vi "myRIO_BRig_RT__Case_Exp_State_initTrial_LC_Sel__v3.vi"(6 "input_dataTrial":u16[][](array[numeric]), 7 "input_spout":enum16{"Left", "Right"}(ring), 8 "input_arrTrig":bool[](array[boolean]), 9 "input_dataBlock":u16[][](array[numeric]), 10 "input_dataLC":u16[](array[numeric]), 11 "input_dataCurrent":u16[](array[numeric])) -> (0 "output_arrTrig":bool[](array[boolean]), 4 "output_dataTrial":u16[][](array[numeric]), 5 "output_dataCurrent":u16[](array[numeric]))   [LabVIEW 2014]
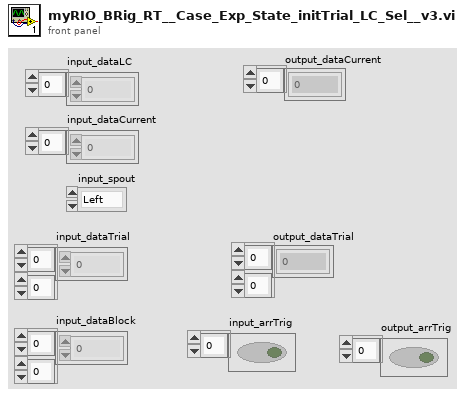
[diagram p1: front panel]
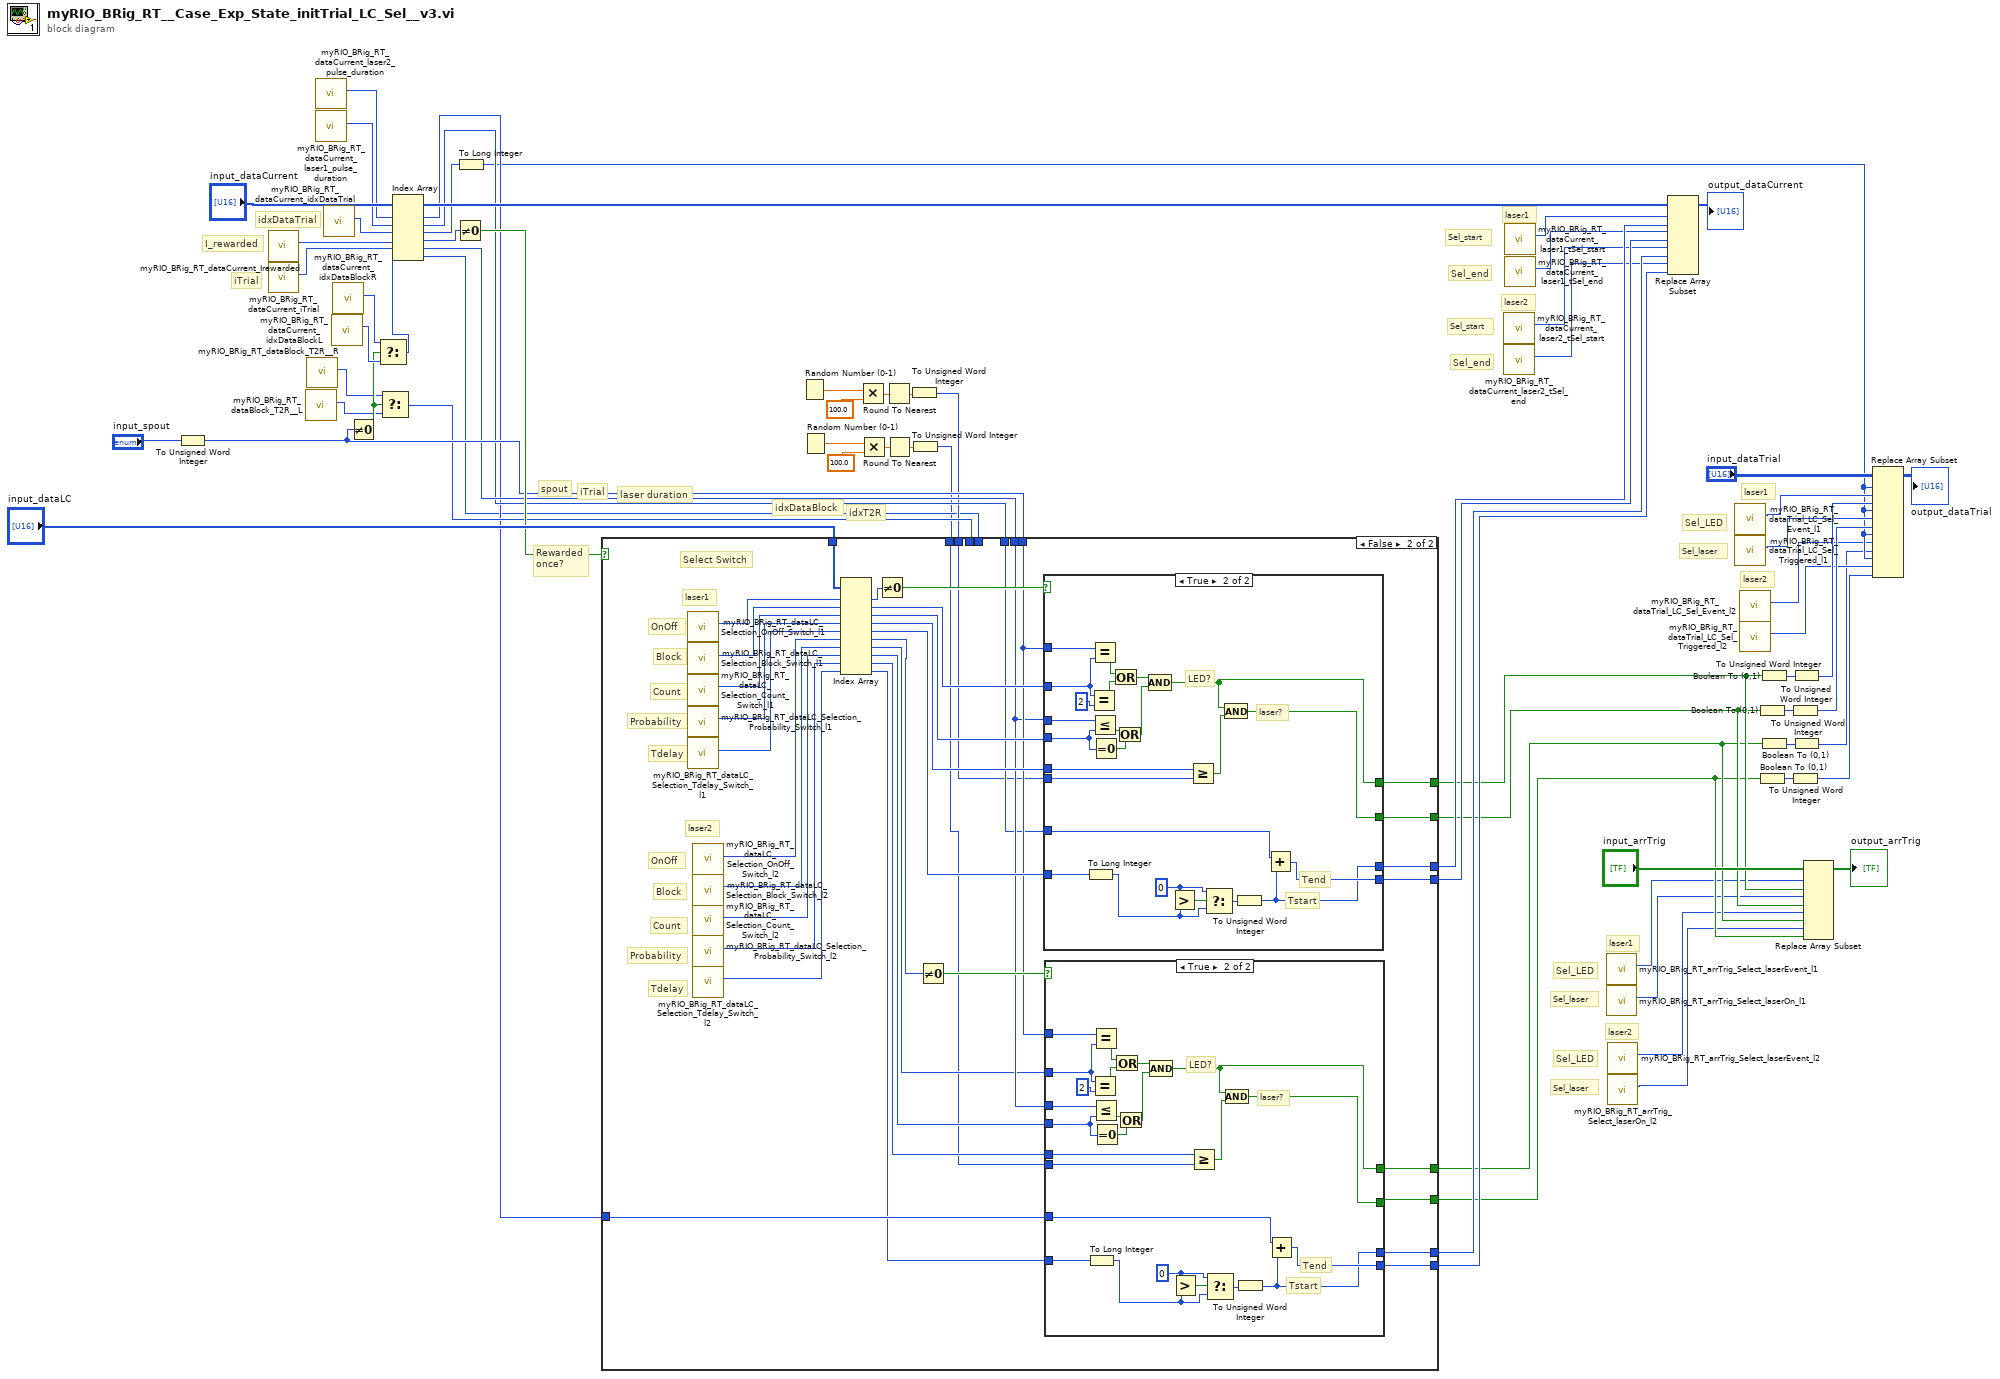
[diagram p0: block diagram]
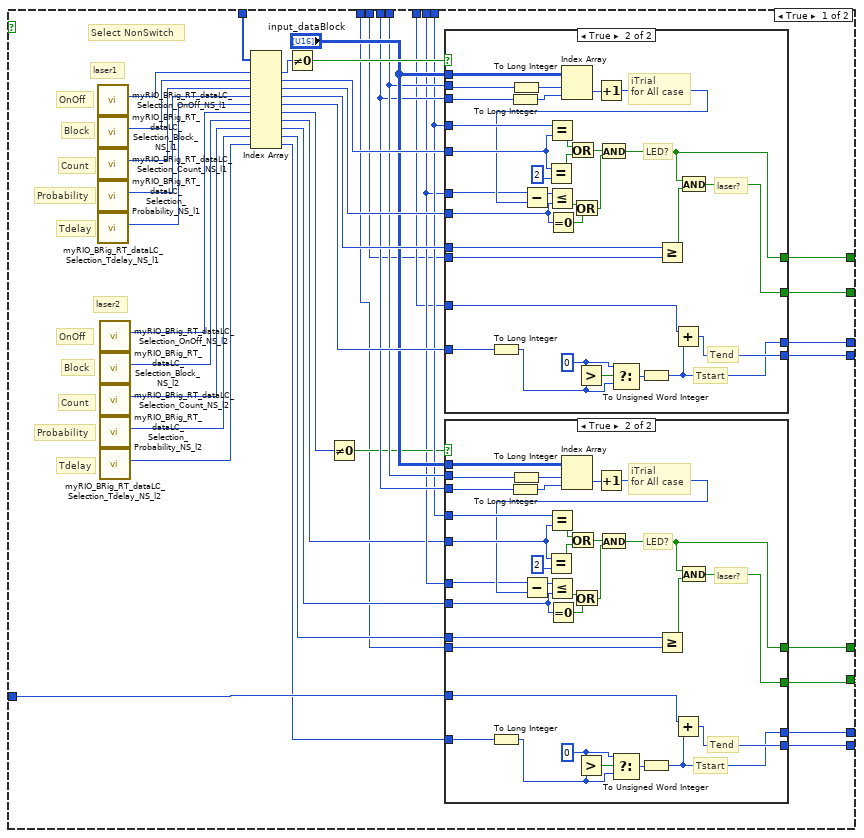
[diagram p2: hidden frame]
diagram:
  # "Sel_LED"
  # "Sel_laser"
  # "Sel_end"
  # "Sel_start"
  # "Sel_LED"
  # "Sel_laser"
  # "Sel_end"
  # "Sel_start"
  # "Sel_LED"
  # "Sel_laser"
  # "laser2"
  # "laser1"
  # "laser2"
  # "laser1"
  # "laser2"
  # "laser1"
  # "idxT2R"
  # "idxDataBlock"
  # "laser duration"
  # "iTrial"
  # "spout"
  # "Rewarded\nonce?"
  # "iTrial"
  # "idxDataTrial"
  # "I_rewarded"
  n1 = To Unsigned Word Integer(number="input_spout") -> (unsigned 16bit integer=w43:u16)
  n2 = call "myRIO_BRig_RT_dataCurrent_Irewarded.vi"() -> ("output_I_rewarded"=w65:i32)  [unwired: 11 in]
  n3 = call "myRIO_BRig_RT_dataCurrent_iTrial.vi"() -> ("output_iTrial"=w54:i32)  [unwired: 11 in]
  n4 = call "myRIO_BRig_RT_dataBlock_T2R__L.vi"() -> ("output_T2R__L"=w49:i32)  [unwired: 11 in]
  n5 = call "myRIO_BRig_RT_dataBlock_T2R__R.vi"() -> ("output_T2R__R"=w50:i32)  [unwired: 11 in]
  n6 = call "myRIO_BRig_RT_dataCurrent_laser2_pulse_duration.vi"() -> ("output_laser2_pulse_duration"=w24:i32)  [unwired: 11 in]
  n7 = call "myRIO_BRig_RT_dataCurrent_laser1_pulse_duration.vi"() -> ("output_laser1_pulse_duration"=w48:i32)  [unwired: 11 in]
  n8 = call "myRIO_BRig_RT_dataCurrent_idxDataTrial.vi"() -> ("output_idxDataTrial"=w58:i32)  [unwired: 11 in]
  n9 = call "myRIO_BRig_RT_dataCurrent_idxDataBlockL.vi"() -> ("output_idxDataBlock__L"=w53:i32)  [unwired: 11 in]
  n10 = call "myRIO_BRig_RT_dataCurrent_idxDataBlockR.vi"() -> ("output_idxDataBlock__R"=w52:i32)  [unwired: 11 in]
  n11 = Not Equal To 0?(x=w43) -> (x != 0?=w51:bool)
  n12 = Select(t=w52, s=w51, f=w53) -> (s? t:f=w21:i32)
  n13 = Select(t=w50, s=w51, f=w49) -> (s? t:f=w40:i32)
  n14 = Index Array(array="input_dataCurrent", index #1=w24, index #2=w48, index #3=w58, index #4=w65, index #5=w54, index #6=w21) -> (element #1=w23:u16, element #2=w41:u16, element #3=w57:u16, element #4=w66:u16, element #5=w42:u16, element #6=w22:u16)
  n15 = Not Equal To 0?(x=w66) -> (x != 0?=w44:bool)
  n16 = To Long Integer(number=w57) -> (32bit integer=w10:i32)
  n17 = Random Number (0-1)() -> (number: 0 to 1=w36:dbl)
  n18 = Random Number (0-1)() -> (number: 0 to 1=w2:dbl)
  n19 = Multiply(x=w36, y=100.0) -> (x*y=w37:dbl)
  n20 = Multiply(x=w2, y=100.0) -> (x*y=w3:dbl)
  n21 = Round To Nearest(number=w37) -> (nearest integer value=w38:dbl)
  n22 = Round To Nearest(number=w3) -> (nearest integer value=w4:dbl)
  n23 = To Unsigned Word Integer(number=w38) -> (unsigned 16bit integer=w35:u16)
  n24 = To Unsigned Word Integer(number=w4) -> (unsigned 16bit integer=w1:u16)
  n25 = case shown="False" w44 {
    tunnel: "input_dataLC" -> [w107 w208]
    tunnel: w43 -> [w97 w192]
    tunnel: w42 -> [w95 w191]
    tunnel: w41 -> [w94 w190]
    tunnel: w22 -> [w99 _]
    tunnel: w40 -> [w98 _]
    tunnel: w35 -> [w68 w172]
    tunnel: [w93 w201] -> w28
    tunnel: [w92 w200] -> w27
    tunnel: [w91 w199] -> w34
    tunnel: [w90 w198] -> w33
    tunnel: [w89 w196] -> w26
    tunnel: [w88 w195] -> w25
    tunnel: [w87 w194] -> w32
    tunnel: [w86 w193] -> w31
    tunnel: w23 -> [w85 w189]
    tunnel: w1 -> [w69 w173]
    frame True {
      # "laser2"
      # "laser1"
      # "Count"
      # "Tdelay"
      # "Probability"
      # "OnOff"
      # "Block"
      # "Count"
      # "Tdelay"
      # "Probability"
      # "OnOff"
      # "Block"
      # "Select NonSwitch"
      n26 = call "myRIO_BRig_RT_dataLC_Selection_OnOff_NS_l1.vi"() -> ("output_Selection_OnOff_NS_l1"=w70:i32)  [unwired: 11 in]
      n27 = call "myRIO_BRig_RT_dataLC_Selection_Block_NS_l1.vi"() -> ("output_Selection_Block_NS_l1"=w71:i32)  [unwired: 11 in]
      n28 = call "myRIO_BRig_RT_dataLC_Selection_Count_NS_l1.vi"() -> ("output_Selection_Count_NS_l1"=w72:i32)  [unwired: 11 in]
      n29 = call "myRIO_BRig_RT_dataLC_Selection_Probability_NS_l1.vi"() -> ("output_Selection_Probability_NS_l1"=w73:i32)  [unwired: 11 in]
      n30 = call "myRIO_BRig_RT_dataLC_Selection_Tdelay_NS_l1.vi"() -> ("output_Selection_Tdelay_NS_l1"=w74:i32)  [unwired: 11 in]
      n31 = call "myRIO_BRig_RT_dataLC_Selection_OnOff_NS_l2.vi"() -> ("output_Selection_OnOff_NS_l2"=w79:i32)  [unwired: 11 in]
      n32 = call "myRIO_BRig_RT_dataLC_Selection_Block_NS_l2.vi"() -> ("output_Selection_Block_NS_l2"=w78:i32)  [unwired: 11 in]
      n33 = call "myRIO_BRig_RT_dataLC_Selection_Count_NS_l2.vi"() -> ("output_Selection_Count_NS_l2"=w77:i32)  [unwired: 11 in]
      n34 = call "myRIO_BRig_RT_dataLC_Selection_Probability_NS_l2.vi"() -> ("output_Selection_Probability_NS_l2"=w76:i32)  [unwired: 11 in]
      n35 = call "myRIO_BRig_RT_dataLC_Selection_Tdelay_NS_l2.vi"() -> ("output_Selection_Tdelay_NS_l2"=w75:i32)  [unwired: 11 in]
      n36 = Index Array(array=w107, index #1=w70, index #2=w71, index #3=w72, index #4=w73, index #5=w74, index #6=w79, index #7=w78, index #8=w77, index #9=w76, index #10=w75) -> (element #1=w103:u16, element #2=w101:u16, element #3=w106:u16, element #4=w105:u16, element #5=w104:u16, element #6=w84:u16, element #7=w83:u16, element #8=w82:u16, element #9=w81:u16, element #10=w80:u16)
      n37 = Not Equal To 0?(x=w103) -> (x != 0?=w102:bool)
      n38 = Not Equal To 0?(x=w84) -> (x != 0?=w96:bool)
      n39 = case shown="True" w102 {
        tunnel: w97 -> [_ w170]
        tunnel: w95 -> [_ w155]
        tunnel: [_ w150] -> w93
        tunnel: [_ w166] -> w92
        tunnel: [_ w146] -> w90
        tunnel: [_ w145] -> w91
        tunnel: w94 -> [_ w144]
        tunnel: w98 -> [_ w161]
        tunnel: w99 -> [_ w163]
        tunnel: w101 -> [_ w158]
        tunnel: w106 -> [_ w157]
        tunnel: w105 -> [_ w153]
        tunnel: w104 -> [_ w143]
        tunnel: "input_dataBlock" -> [_ w142]
        tunnel: w68 -> [_ w141]
        frame False {
        }
        frame True {
          w148 = 0 ("x")
          # "Tstart"
          # "Tend"
          # "iTrial\nfor All case"
          # "laser?"
          # "LED?"
          n40 = To Long Integer(number=w143) -> (32bit integer=w140:i32)
          n41 = To Long Integer(number=w161) -> (32bit integer=w160:i32)
          n42 = To Long Integer(number=w163) -> (32bit integer=w162:i32)
          n43 = Equal?(x=w158, y=u16 2) -> (x = y?=w168:bool)
          n44 = Equal?(x=w170, y=w158) -> (x = y?=w169:bool)
          n45 = Equal To 0?(x=w157) -> (x = 0?=w164:bool)
          n46 = Index Array(array=w142, index (row)=w162, index (col)=w160) -> (element=w159:u16)
          n47 = Or(x=w169, y=w168) -> (x .or. y?=w152:bool)
          n48 = Greater?(x=w148, y=w140) -> (0:w147:bool)
          n49 = Increment(x=w159) -> (x+1=w156:u16)
          n50 = Subtract(x=w155, y=w156) -> (x-y=w154:u16)
          n51 = Less Or Equal?(x=w154, y=w157) -> (x <= y?=w165:bool)
          n52 = Or(x=w165, y=w164) -> (x .or. y?=w151:bool)
          n53 = And(x=w152, y=w151) -> (x .and. y?=w150:bool)
          n54 = Select(t=w148, s=w147, f=w140) -> (s? t:f=w149:i32)
          n55 = To Unsigned Word Integer(number=w149) -> (unsigned 16bit integer=w145:u16)
          n56 = Greater Or Equal?(x=w153, y=w141) -> (x >= y?=w167:bool)
          n57 = Add(x=w144, y=w145) -> (x+y=w146:u16)
          n58 = And(x=w150, y=w167) -> (x .and. y?=w166:bool)
        }
      }
      n59 = case shown="True" w96 {
        tunnel: w97 -> [_ w138]
        tunnel: w95 -> [_ w123]
        tunnel: [_ w118] -> w89
        tunnel: [_ w134] -> w88
        tunnel: [_ w114] -> w86
        tunnel: [_ w113] -> w87
        tunnel: w85 -> [_ w112]
        tunnel: w98 -> [_ w129]
        tunnel: w99 -> [_ w131]
        tunnel: w83 -> [_ w126]
        tunnel: w82 -> [_ w125]
        tunnel: w81 -> [_ w121]
        tunnel: w80 -> [_ w111]
        tunnel: "input_dataBlock" -> [_ w110]
        tunnel: w69 -> [_ w109]
        frame False {
        }
        frame True {
          w116 = 0 ("x")
          # "Tstart"
          # "Tend"
          # "iTrial\nfor All case"
          # "laser?"
          # "LED?"
          n60 = To Long Integer(number=w111) -> (32bit integer=w108:i32)
          n61 = To Long Integer(number=w129) -> (32bit integer=w128:i32)
          n62 = To Long Integer(number=w131) -> (32bit integer=w130:i32)
          n63 = Equal?(x=w126, y=u16 2) -> (x = y?=w136:bool)
          n64 = Equal?(x=w138, y=w126) -> (x = y?=w137:bool)
          n65 = Equal To 0?(x=w125) -> (x = 0?=w132:bool)
          n66 = Index Array(array=w110, index (row)=w130, index (col)=w128) -> (element=w127:u16)
          n67 = Or(x=w137, y=w136) -> (x .or. y?=w120:bool)
          n68 = Greater?(x=w116, y=w108) -> (0:w115:bool)
          n69 = Increment(x=w127) -> (x+1=w124:u16)
          n70 = Subtract(x=w123, y=w124) -> (x-y=w122:u16)
          n71 = Less Or Equal?(x=w122, y=w125) -> (x <= y?=w133:bool)
          n72 = Or(x=w133, y=w132) -> (x .or. y?=w119:bool)
          n73 = And(x=w120, y=w119) -> (x .and. y?=w118:bool)
          n74 = Select(t=w116, s=w115, f=w108) -> (s? t:f=w117:i32)
          n75 = To Unsigned Word Integer(number=w117) -> (unsigned 16bit integer=w113:u16)
          n76 = Greater Or Equal?(x=w121, y=w109) -> (x >= y?=w135:bool)
          n77 = Add(x=w112, y=w113) -> (x+y=w114:u16)
          n78 = And(x=w118, y=w135) -> (x .and. y?=w134:bool)
        }
      }
    }
    frame False {
      # "laser2"
      # "laser1"
      # "Count"
      # "Tdelay"
      # "Probability"
      # "OnOff"
      # "Block"
      # "Count"
      # "Tdelay"
      # "Probability"
      # "OnOff"
      # "Block"
      # "Select Switch"
      n79 = call "myRIO_BRig_RT_dataLC_Selection_OnOff_Switch_l1.vi"() -> ("output_Selection_OnOff_Switch_l1"=w188:i32)  [unwired: 11 in]
      n80 = call "myRIO_BRig_RT_dataLC_Selection_Block_Switch_l1.vi"() -> ("output_Selection_Block_Switch_l1"=w187:i32)  [unwired: 11 in]
      n81 = call "myRIO_BRig_RT_dataLC_Selection_Count_Switch_l1.vi"() -> ("output_Selection_Count_Switch_l1"=w186:i32)  [unwired: 11 in]
      n82 = call "myRIO_BRig_RT_dataLC_Selection_Probability_Switch_l1.vi"() -> ("output_Selection_Probability_Switch_l1"=w185:i32)  [unwired: 11 in]
      n83 = call "myRIO_BRig_RT_dataLC_Selection_Tdelay_Switch_l1.vi"() -> ("output_Selection_Tdelay_Switch_l1"=w184:i32)  [unwired: 11 in]
      n84 = call "myRIO_BRig_RT_dataLC_Selection_OnOff_Switch_l2.vi"() -> ("output_Selection_OnOff_Switch_l2"=w174:i32)  [unwired: 11 in]
      n85 = call "myRIO_BRig_RT_dataLC_Selection_Block_Switch_l2.vi"() -> ("output_Selection_Block_Switch_l2"=w175:i32)  [unwired: 11 in]
      n86 = call "myRIO_BRig_RT_dataLC_Selection_Count_Switch_l2.vi"() -> ("output_Selection_Count_Switch_l2"=w176:i32)  [unwired: 11 in]
      n87 = call "myRIO_BRig_RT_dataLC_Selection_Probability_Switch_l2.vi"() -> ("output_Selection_Probability_Switch_l1"=w177:i32)  [unwired: 11 in]
      n88 = call "myRIO_BRig_RT_dataLC_Selection_Tdelay_Switch_l2.vi"() -> ("output_Selection_Tdelay_Switch_l2"=w178:i32)  [unwired: 11 in]
      n89 = Index Array(array=w208, index #1=w188, index #2=w187, index #3=w186, index #4=w185, index #5=w184, index #6=w174, index #7=w175, index #8=w176, index #9=w177, index #10=w178) -> (element #1=w207:u16, element #2=w204:u16, element #3=w203:u16, element #4=w205:u16, element #5=w202:u16, element #6=w183:u16, element #7=w182:u16, element #8=w181:u16, element #9=w180:u16, element #10=w179:u16)
      n90 = Not Equal To 0?(x=w207) -> (x != 0?=w206:bool)
      n91 = Not Equal To 0?(x=w183) -> (x != 0?=w197:bool)
      n92 = case shown="True" w206 {
        tunnel: w192 -> [_ w255]
        tunnel: w204 -> [_ w254]
        tunnel: w191 -> [_ w253]
        tunnel: [_ w248] -> w201
        tunnel: [_ w247] -> w200
        tunnel: [_ w237] -> w198
        tunnel: w202 -> [_ w239]
        tunnel: [_ w236] -> w199
        tunnel: w203 -> [_ w246]
        tunnel: w190 -> [_ w238]
        tunnel: w172 -> [_ w235]
        tunnel: w205 -> [_ w234]
        frame False {
        }
        frame True {
          w241 = 0 ("x")
          # "Tstart"
          # "Tend"
          # "laser?"
          # "LED?"
          n93 = To Long Integer(number=w239) -> (32bit integer=w233:i32)
          n94 = Equal?(x=w254, y=u16 2) -> (x = y?=w251:bool)
          n95 = Equal?(x=w255, y=w254) -> (x = y?=w252:bool)
          n96 = Less Or Equal?(x=w253, y=w246) -> (x <= y?=w245:bool)
          n97 = Equal To 0?(x=w246) -> (x = 0?=w244:bool)
          n98 = Or(x=w252, y=w251) -> (x .or. y?=w250:bool)
          n99 = Or(x=w245, y=w244) -> (x .or. y?=w243:bool)
          n100 = Compound Arithmetic op=AND(w250, w243) -> (w248:bool)
          n101 = Greater?(x=w241, y=w233) -> (0:w240:bool)
          n102 = Greater Or Equal?(x=w234, y=w235) -> (x >= y?=w249:bool)
          n103 = Select(t=w241, s=w240, f=w233) -> (s? t:f=w242:i32)
          n104 = And(x=w248, y=w249) -> (x .and. y?=w247:bool)
          n105 = To Unsigned Word Integer(number=w242) -> (unsigned 16bit integer=w236:u16)
          n106 = Add(x=w238, y=w236) -> (x+y=w237:u16)
        }
      }
      n107 = case shown="True" w197 {
        tunnel: w192 -> [_ w231]
        tunnel: w182 -> [_ w230]
        tunnel: w191 -> [_ w229]
        tunnel: [_ w224] -> w196
        tunnel: [_ w223] -> w195
        tunnel: [_ w213] -> w193
        tunnel: w179 -> [_ w215]
        tunnel: [_ w212] -> w194
        tunnel: w181 -> [_ w222]
        tunnel: w189 -> [_ w214]
        tunnel: w173 -> [_ w211]
        tunnel: w180 -> [_ w210]
        frame False {
        }
        frame True {
          w217 = 0 ("x")
          # "Tstart"
          # "Tend"
          # "laser?"
          # "LED?"
          n108 = To Long Integer(number=w215) -> (32bit integer=w209:i32)
          n109 = Equal?(x=w230, y=u16 2) -> (x = y?=w227:bool)
          n110 = Equal?(x=w231, y=w230) -> (x = y?=w228:bool)
          n111 = Less Or Equal?(x=w229, y=w222) -> (x <= y?=w221:bool)
          n112 = Equal To 0?(x=w222) -> (x = 0?=w220:bool)
          n113 = Or(x=w228, y=w227) -> (x .or. y?=w226:bool)
          n114 = Or(x=w221, y=w220) -> (x .or. y?=w219:bool)
          n115 = Compound Arithmetic op=AND(w226, w219) -> (w224:bool)
          n116 = Greater?(x=w217, y=w209) -> (0:w216:bool)
          n117 = Greater Or Equal?(x=w210, y=w211) -> (x >= y?=w225:bool)
          n118 = Select(t=w217, s=w216, f=w209) -> (s? t:f=w218:i32)
          n119 = And(x=w224, y=w225) -> (x .and. y?=w223:bool)
          n120 = To Unsigned Word Integer(number=w218) -> (unsigned 16bit integer=w212:u16)
          n121 = Add(x=w214, y=w212) -> (x+y=w213:u16)
        }
      }
    }
  }
  n122 = call "myRIO_BRig_RT_dataCurrent_laser2_tSel_start.vi"() -> ("output_laser2_tSel_start"=w18:i32)  [unwired: 11 in]
  n123 = call "myRIO_BRig_RT_dataCurrent_laser2_tSel_end.vi"() -> ("output_laser2_tSel_end"=w17:i32)  [unwired: 11 in]
  n124 = call "myRIO_BRig_RT_dataCurrent_laser1_tSel_start.vi"() -> ("output_laser1_tSel_start"=w19:i32)  [unwired: 11 in]
  n125 = call "myRIO_BRig_RT_dataCurrent_laser1_tSel_end.vi"() -> ("output_laser1_tSel_end"=w20:i32)  [unwired: 11 in]
  n126 = call "myRIO_BRig_RT_arrTrig_Select_laserEvent_l1.vi"() -> ("output_arrTrig_Select_laserEvent_l1"=w15:i32)  [unwired: 11 in]
  n127 = call "myRIO_BRig_RT_arrTrig_Select_laserOn_l1.vi"() -> ("output_arrTrig_Select_laserOn_l1"=w16:i32)  [unwired: 11 in]
  n128 = call "myRIO_BRig_RT_arrTrig_Select_laserEvent_l2.vi"() -> ("output_arrTrig_Select_laserEvent_l2"=w14:i32)  [unwired: 11 in]
  n129 = call "myRIO_BRig_RT_arrTrig_Select_laserOn_l2.vi"() -> ("output_arrTrig_Select_laserOn_l2"=w13:i32)  [unwired: 11 in]
  n130 = Replace Array Subset(array="input_dataCurrent", new element #1=w34, index #1=w19, new element #2=w33, index #2=w20, new element #3=w32, index #3=w18, new element #4=w31, index #4=w17) -> (→"output_dataCurrent":u16[])
  n131 = call "myRIO_BRig_RT_dataTrial_LC_Sel_Event_l1.vi"() -> ("output_LC_Sel_Event_l1"=w11:i32)  [unwired: 11 in]
  n132 = call "myRIO_BRig_RT_dataTrial_LC_Sel_Triggered_l1.vi"() -> ("output_LC_Sel_Triggered_l1"=w12:i32)  [unwired: 11 in]
  n133 = call "myRIO_BRig_RT_dataTrial_LC_Sel_Event_l2.vi"() -> ("output_LC_Sel_Event_l2"=w9:i32)  [unwired: 11 in]
  n134 = call "myRIO_BRig_RT_dataTrial_LC_Sel_Triggered_l2.vi"() -> ("output_LC_Sel_Triggered_l2"=w8:i32)  [unwired: 11 in]
  n135 = Boolean To (0,1)(Boolean=w27) -> (0, 1=w61:i16)
  n136 = Boolean To (0,1)(Boolean=w25) -> (0, 1=w30:i16)
  n137 = Boolean To (0,1)(Boolean=w28) -> (0, 1=w62:i16)
  n138 = Boolean To (0,1)(Boolean=w26) -> (0, 1=w29:i16)
  n139 = To Unsigned Word Integer(number=w61) -> (unsigned 16bit integer=w55:u16)
  n140 = To Unsigned Word Integer(number=w30) -> (unsigned 16bit integer=w6:u16)
  n141 = To Unsigned Word Integer(number=w62) -> (unsigned 16bit integer=w56:u16)
  n142 = To Unsigned Word Integer(number=w29) -> (unsigned 16bit integer=w7:u16)
  n143 = Replace Array Subset(array="input_arrTrig", new element #1=w28, index #1=w15, new element #2=w27, index #2=w16, new element #3=w26, index #3=w14, new element #4=w25, index #4=w13) -> (→"output_arrTrig":bool[])
  n144 = Replace Array Subset(array="input_dataTrial", new element #1=w56, index (row) #1=w10, index (col) #1=w11, new element #2=w55, index (row) #2=w10, index (col) #2=w12, new element #3=w7, index (row) #3=w10, index (col) #3=w9, new element #4=w6, index (row) #4=w10, index (col) #4=w8) -> (→"output_dataTrial":u16[][])
